vi "To Image.vi"(8 "error in (no error)":errorcluster, 11 "Canvas in":refnum<class "Drawer .Net.lvclass">) -> (0 "error out":errorcluster, 2 "Bitmap":u32[][](array[numeric]), 3 "Canvas out":refnum<class "Drawer .Net.lvclass">)   [LabVIEW 2020, in "Glyph .NET.lvlib" / "Drawer .Net.lvclass"]
uses:
  Drawer .Net.lvclass
  Drawer .Net.lvclass/Drawer .Net.ctl
  System.Drawing
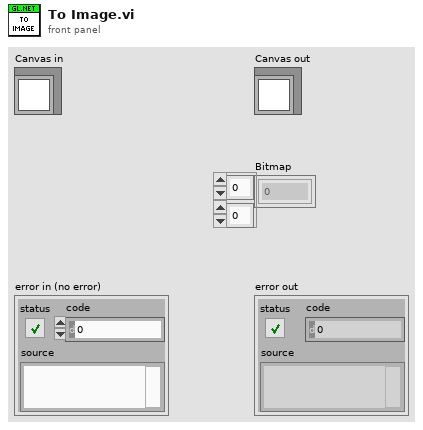
[diagram p1: front panel]
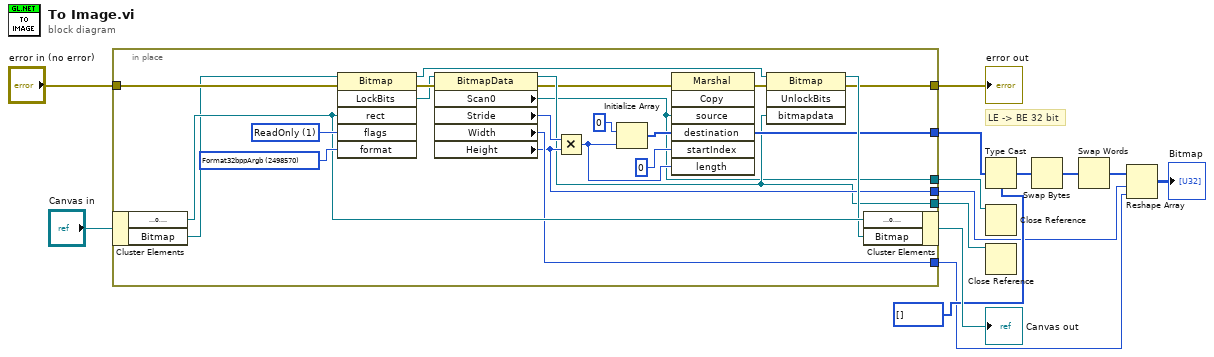
[diagram p0: block diagram]
diagram:
  # "LE -> BE 32 bit"
  n1 = in-place {
    in-place-border: "error in (no error)" -> [w32]
    in-place-border: [w21] -> w1
    in-place-border: [w20] -> w2
    in-place-border: [w15] -> w11
    in-place-border: [w25] -> w7
    in-place-border: [w19] -> w10
    in-place-border: [w18] -> w9
    w30 = 2498570 items=["DontCare, Undefined"=0, "Max"=15, "Indexed"=65536, "Gdi"=131072, "Format16bppRgb555"=135173, "Format16bppRgb565"=135174, "Format24bppRgb"=137224, "Format32bppRgb"=139273, "Format1bppIndexed"=196865, "Format4bppIndexed"=197634, "Format8bppIndexed"=198659, "Alpha"=262144, "Format16bppArgb1555"=397319, "PAlpha"=524288, "Format32bppPArgb"=925707, "Extended"=1048576, "Format16bppGrayScale"=1052676, "Format48bppRgb"=1060876, "Format64bppPArgb"=1851406, "Canonical"=2097152, "Format32bppArgb"=2498570, "Format64bppArgb"=3424269] ("format")
    w31 = 1 items=["ReadOnly"=1, "WriteOnly"=2, "ReadWrite"=3, "UserInputBuffer"=4] ("flags")
    n2 = in-place-cluster #1("Canvas in") -> ("Rectangle"=w28:refnum<k24>, "Bitmap"=w27:refnum<k24>)
    n3 = invoke class="Bitmap" method="LockBits"(reference=w27, error in=w32, "rect"=w28, "flags"=w31, "format"=w30) -> (reference out=w33:refnum<k24>, error out=w36:errorcluster, "LockBits"=w35:refnum<k24>)  [unwired: 1 in, 3 out]
    n4 = property class="BitmapData"(reference=w35, error in=w36) -> (reference out=w19:refnum<k24>, error out=w17:errorcluster, "Scan0"=w18:refnum<k24>, "Stride"=w34:i32, "Width"=w21:i32, "Height"=w20:i32)
    n5 = Multiply(x=w34, y=w20) -> (x*y=w29:i32)
    n6 = Initialize Array(u8 0, w29) -> (w22:u8[])
    n7 = invoke class="Marshal" method="Copy"(error in=w17, "source"=w18, "destination"=w22, "startIndex"=0, "length"=w29) -> (error out=w16:errorcluster, "destination"=w25:u8[])  [unwired: 2 in, 5 out]
    n8 = invoke class="Bitmap" method="UnlockBits"(reference=w33, error in=w16, "bitmapdata"=w19) -> (reference out=w26:refnum<k24>, error out=w15:errorcluster)  [unwired: 1 in, 2 out]
    n9 = in-place-cluster #1("Rectangle"=w28, "Bitmap"=w26) -> (→"Canvas out":refnum<class "Drawer .Net.lvclass">)
  }
  "error out" <- w11
  n10 = Type Cast(type=u32[] [], x=w7) -> (*(type *) &x=w6:u32[])
  n11 = Close Reference(reference=w9) -> ()  [unwired: 1 in, 1 out]
  n12 = Close Reference(reference=w10) -> ()  [unwired: 1 in, 1 out]
  n13 = Swap Bytes(anything=w6) -> (byte swapped=w4:u32[])
  n14 = Swap Words(1:w4) -> (0:w3:u32[])
  n15 = Reshape Array(w3, w2, w1) -> (→"Bitmap":u32[][])
